vi "VI_InLibrary.vi"(11 "Input String":string) -> (3 "Output String":string)   [LabVIEW 2012, in "LabVIEW_Library.lvlib"]
uses:
  LabVIEW_Library.lvlib
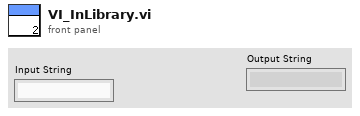
[diagram p1: front panel]
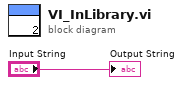
[diagram p0: block diagram]
diagram:
  "Output String" <- "Input String"
